vi "ClimbExecute_SIM.vi"(8 "error in (no error)":errorcluster, 11 "Inputs":T3) -> (0 "error out":errorcluster, 2 "InfoOutput":T1, 3 "Outputs":T2)   [LabVIEW 2023]
uses:
  <vilib>/Rock Robotics/WPI/ThirdParty/JAS_Junk/TrajLib/Timer_New.vi
  <vilib>/Rock Robotics/WPI/ThirdParty/JAS_Junk/TrajLib/VI/BoolCmd_Recv_Internal.vi
  <vilib>/Rock Robotics/WPI/ThirdParty/JAS_Junk/TrajLib/VI/BoolCmd_ObtainQueue.vi
  <vilib>/Rock Robotics/Network Tables/NT Write Number.vi
  <vilib>/Utility/semaphor.llb/Obtain Semaphore Reference.vi
  <vilib>/Rock Robotics/WPI/ThirdParty/JAS_Junk/TrajLib/Timer_Reset.vi
  <vilib>/Rock Robotics/WPI/ThirdParty/JAS_Junk/TrajLib/Timer_Start.vi
  <vilib>/Rock Robotics/WPI/ThirdParty/JAS_Junk/TrajLib/Timer_Stop.vi
  <vilib>/Rock Robotics/WPI/ThirdParty/JAS_Junk/TrajLib/Timer_HasPeriodPassedOnce.vi
  <vilib>/Rock Robotics/Network Tables/NT Write Boolean.vi
  <vilib>/Rock Robotics/WPI/ThirdParty/JAS_Junk/TrajLib/Trajectory_Library.lvlib
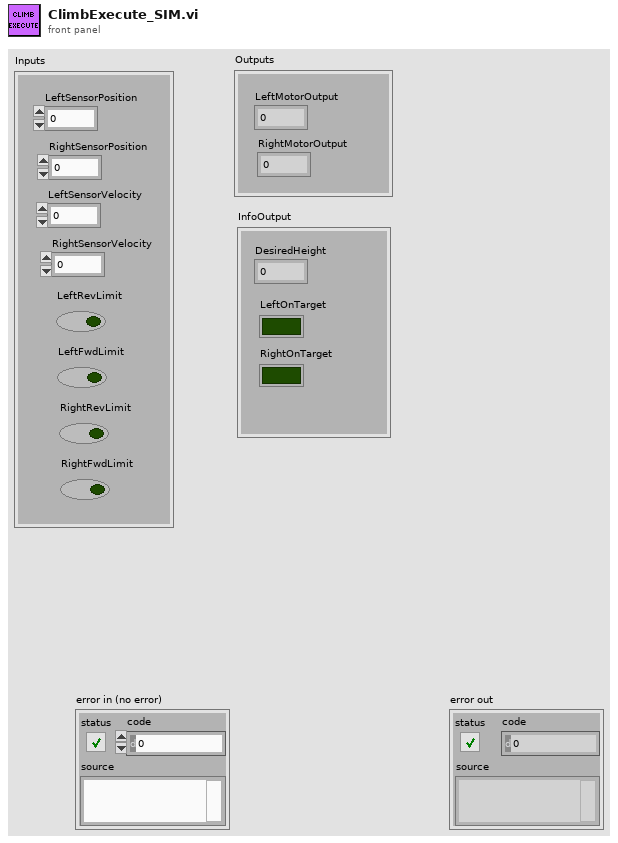
[diagram p1: front panel]
types:
  T1 = cluster{"DesiredHeight":dbl, "LeftOnTarget":bool, "RightOnTarget":bool}
  T2 = cluster{"LeftMotorOutput":dbl, "RightMotorOutput":dbl}
  T3 = cluster{"LeftSensorPosition":dbl, "RightSensorPosition":dbl, "LeftSensorVelocity":dbl, "RightSensorVelocity":dbl, "LeftRevLimit":bool, "LeftFwdLimit":bool, "RightRevLimit":bool, "RightFwdLimit":bool}
  T4 = typedef "Trajectory_Library.lvlib/PosCtrl_Tuning_Type.ctl" = cluster{"Slope":dbl, "Offset":dbl, "Error Deadband":dbl, "At Reference Count":i32, "Negate Output":bool, "Max Allowd Position":dbl, "Min Allowd Position":dbl}
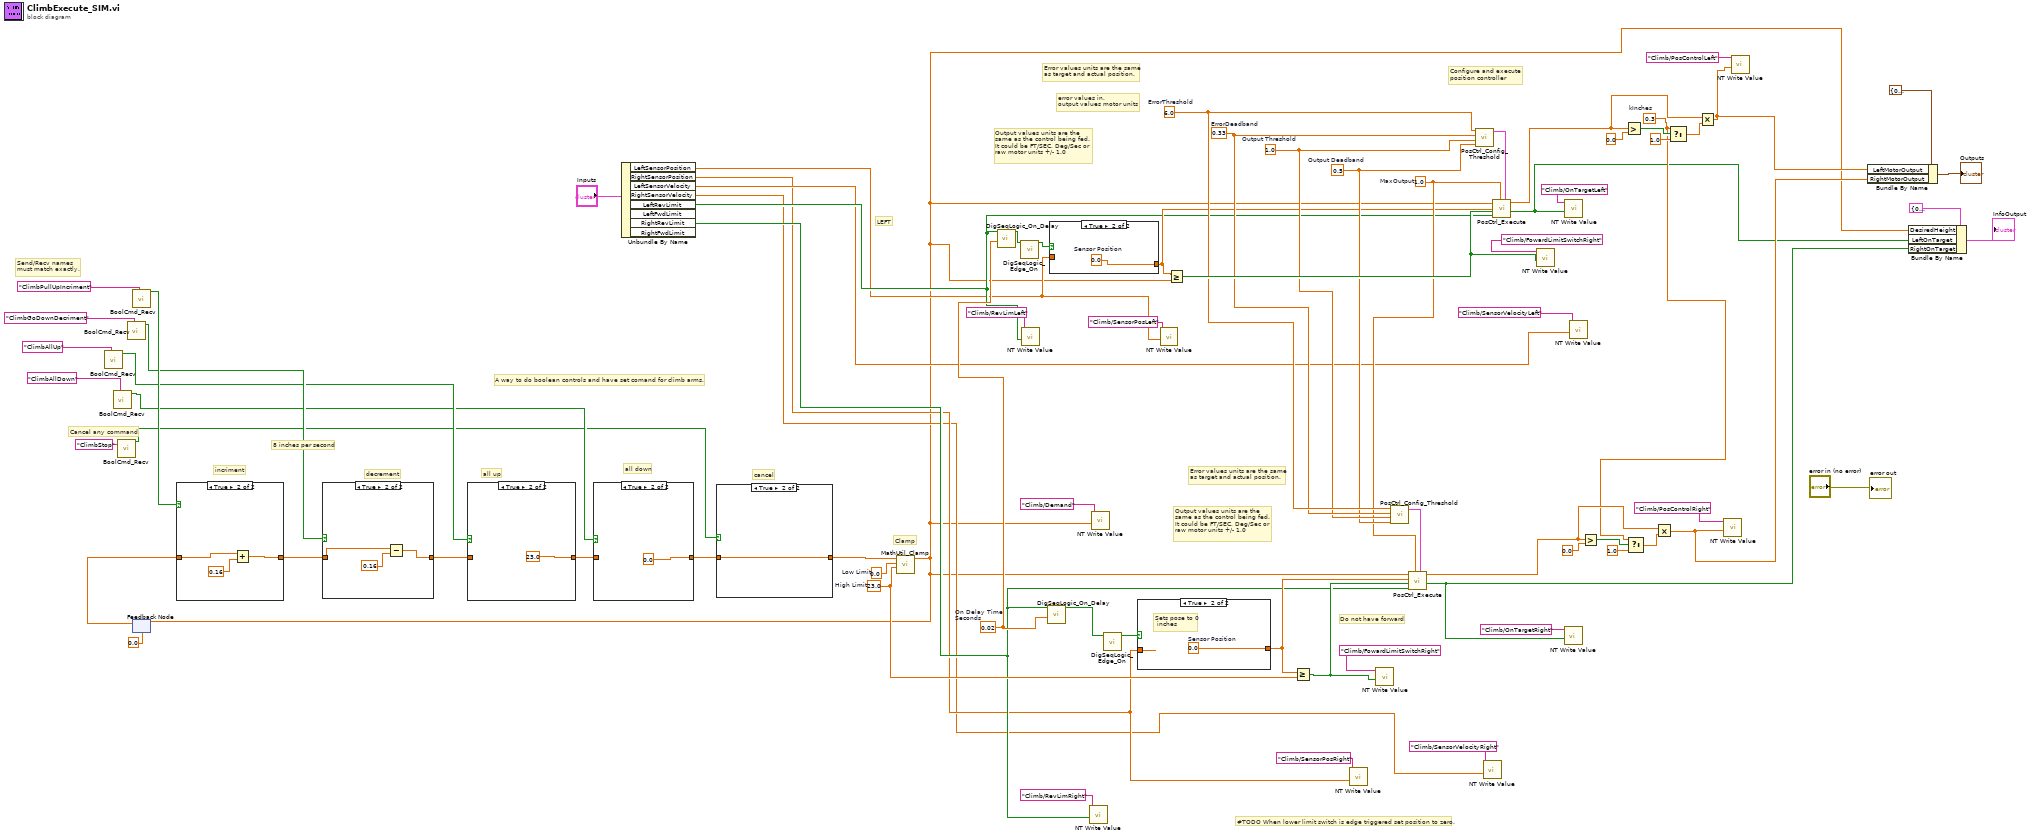
[diagram p0: block diagram]
diagram:
  w17 = 0.3  # kInches
  w32 = 0.02  # On Delay Time Seconds
  w45 = 23.0  # High Limit
  w54 = 0.0  # Low Limit
  w34 = 1.0  # MaxOutput
  w38 = 6.0  # ErrorThreshold
  w37 = 0.33  # ErrorDeadband
  w36 = 1.0  # Output Threshold
  w35 = 0.5  # Output Deadband
  # "LEFT"
  # "#TODO When lower limit switch is edge triggered set position to zero."
  # "cancel"
  # "Clamp"
  # "8 inches per second"
  # "all down"
  # "all up"
  # "decrement"
  # "incriment"
  # "Cancel any command"
  # "Send/Recv names\nmust match exactly."
  # "A way to do boolean controls and have set comand for climb arms."
  # "error values in.\noutput values motor units"
  # "Do not have forward"
  # "Output values units are the\nsame as the control being fed.  \nIt could be FT/SEC, Deg/Sec or\nraw motor units +/- 1.0"
  # "Error values units are the same \nas target and actual position."
  # "Output values units are the\nsame as the control being fed.  \nIt could be FT/SEC, Deg/Sec or\nraw motor units +/- 1.0"
  # "Error values units are the same \nas target and actual position."
  # "Configure and execute \nposition controller"
  n1 = call <vilib>:"BoolCmd_Recv.vi"("Command Name"="ClimbAllUp") -> ("New Request"=w49:bool)  [unwired: 9 in, 1 out]
  n2 = call <vilib>:"BoolCmd_Recv.vi"("Command Name"="ClimbAllDown") -> ("New Request"=w48:bool)  [unwired: 9 in, 1 out]
  n3 = call <vilib>:"BoolCmd_Recv.vi"("Command Name"="ClimbStop") -> ("New Request"=w47:bool)  [unwired: 9 in, 1 out]
  n4 = call <vilib>:"BoolCmd_Recv.vi"("Command Name"="ClimbGoDownDecriment") -> ("New Request"=w50:bool)  [unwired: 9 in, 1 out]
  n5 = call <vilib>:"BoolCmd_Recv.vi"("Command Name"="ClimbPullUpIncriment") -> ("New Request"=w51:bool)  [unwired: 9 in, 1 out]
  n6 = feedback #1(0.0 ("false")) -> (w58:dbl)
  n7 = case shown="True" w51 {
    tunnel: w58 -> [w77 w80]
    tunnel: [w77 w78] -> w57
    frame False {
    }
    frame True {
      n8 = Add(x=w80, y=0.16) -> (x+y=w78:dbl)
    }
  }
  n9 = case shown="True" w50 {
    tunnel: w57 -> [w81 w83]
    tunnel: [w81 w82] -> w56
    frame False {
    }
    frame True {
      n10 = Subtract(x=w83, y=0.16) -> (x-y=w82:dbl)
    }
  }
  n11 = case shown="True" w49 {
    tunnel: w56 -> [w85 _]
    tunnel: [w85 23.0 ("y")] -> w55
    frame False {
    }
    frame True {
    }
  }
  n12 = case shown="True" w48 {
    tunnel: w55 -> [w87 _]
    tunnel: [w87 0.0 ("y")] -> w53
    frame False {
    }
    frame True {
    }
  }
  n13 = Unbundle By Name("Inputs") -> ("LeftSensorPosition"=w14:dbl, "RightSensorPosition"=w8:dbl, "LeftSensorVelocity"=w13:dbl, "RightSensorVelocity"=w7:dbl, "LeftRevLimit"=w15:bool, "RightRevLimit"=w9:bool)  [unwired: 2 out]
  n14 = case shown="True" w47 {
    tunnel: w53 -> [w89 w90]
    tunnel: [w89 w90] -> w52
    frame False {
    }
    frame True {
    }
  }
  n15 = call <vilib>:"MathUtil_Clamp.vi"("High Limit"=w45, "Low Limit"=w54, "Value"=w52) -> ("Result"=w1:dbl)  [unwired: 8 in]
  n16 = feedback-in #1(w1) -> ()
  n17 = call <vilib>:"DigSeqLogic_On_Delay.vi"("Delay"=w32, "Input"=w15) -> ("Output"=w31:bool)  [unwired: 8 in, 1 out]
  n18 = call <vilib>:"DigSeqLogic_Edge_On.vi"("Input"=w31) -> ("On Edge"=w30:bool)  [unwired: 10 in]
  n19 = call-poly <vilib>:"NT Write Value.vi"("value"=w15, "name"="Climb/RevLimLeft") -> ()  [unwired: 9 in, 1 out]
  n20 = call <vilib>:"DigSeqLogic_On_Delay.vi"("Delay"=w32, "Input"=w9) -> ("Output"=w40:bool)  [unwired: 8 in, 1 out]
  n21 = case shown="True" w30 {
    tunnel: w14 -> [w91 _]
    tunnel: [w91 w92] -> w29
    frame False {
    }
    frame True {
      w92 = 0.0  # Sensor Position
    }
  }
  n22 = call-poly <vilib>:"NT Write Value.vi"("value"=w9, "name"="Climb/RevLimRight") -> ()  [unwired: 9 in, 1 out]
  n23 = call-poly <vilib>:"NT Write Value.vi"("value"=w1, "name"="Climb/Demand") -> ()  [unwired: 9 in, 1 out]
  n24 = call <vilib>:"DigSeqLogic_Edge_On.vi"("Input"=w40) -> ("On Edge"=w33:bool)  [unwired: 10 in]
  n25 = case shown="True" w33 {
    tunnel: w8 -> [w93 _]
    tunnel: [w93 w94] -> w39
    frame False {
    }
    frame True {
      w94 = 0.0  # Sensor Position
      # "Sets pose to 0\n inches"
    }
  }
  n26 = call-poly <vilib>:"NT Write Value.vi"("value"=w14, "name"="Climb/SensorPosLeft") -> ()  [unwired: 9 in, 1 out]
  n27 = Greater Or Equal?(x=w29, y=w1) -> (x >= y?=w41:bool)
  n28 = Greater Or Equal?(x=w39, y=w45) -> (x >= y?=w43:bool)
  n29 = call-poly <vilib>:"NT Write Value.vi"("value"=w8, "name"="Climb/SensorPosRight") -> ()  [unwired: 9 in, 1 out]
  n30 = call-poly <vilib>:"NT Write Value.vi"("value"=w43, "name"="Climb/FowardLimitSwitchRight") -> ()  [unwired: 9 in, 1 out]
  n31 = call <vilib>:"PosCtrl_Config_Threshold.vi"("Output Deadband"=w35, "Output Threshold"=w36, "ErrorDeadband"=w37, "ErrorThreshold"=w38) -> ("PosCtrl_Config_Params"=w66:T4)  [unwired: 7 in]
  n32 = call <vilib>:"PosCtrl_Execute.vi"("PosCtrl_Config_Params"=w66, "MaxOutput"=w34, "Rev Limit Switch"=w9, "Fwd Limit Switch"=w43, "CurrentPosition"=w39, "TargetPosition"=w1) -> ("OnTarget"=w2:bool, "Output"=w18:dbl)  [unwired: 3 in, 1 out]
  n33 = call <vilib>:"PosCtrl_Config_Threshold.vi"("Output Deadband"=w35, "Output Threshold"=w36, "ErrorDeadband"=w37, "ErrorThreshold"=w38) -> ("PosCtrl_Config_Params"=w76:T4)  [unwired: 7 in]
  n34 = call-poly <vilib>:"NT Write Value.vi"("value"=w7, "name"="Climb/SensorVelocityRight") -> ()  [unwired: 9 in, 1 out]
  n35 = call <vilib>:"PosCtrl_Execute.vi"("PosCtrl_Config_Params"=w76, "MaxOutput"=w34, "Rev Limit Switch"=w15, "Fwd Limit Switch"=w41, "CurrentPosition"=w29, "TargetPosition"=w1) -> ("OnTarget"=w3:bool, "Output"=w24:dbl)  [unwired: 3 in, 1 out]
  n36 = call-poly <vilib>:"NT Write Value.vi"("value"=w41, "name"="Climb/FowardLimitSwitchRight") -> ()  [unwired: 9 in, 1 out]
  n37 = call-poly <vilib>:"NT Write Value.vi"("value"=w2, "name"="Climb/OnTargetRight") -> ()  [unwired: 9 in, 1 out]
  n38 = call-poly <vilib>:"NT Write Value.vi"("value"=w3, "name"="Climb/OnTargetLeft") -> ()  [unwired: 9 in, 1 out]
  n39 = call-poly <vilib>:"NT Write Value.vi"("value"=w13, "name"="Climb/SensorVelocityLeft") -> ()  [unwired: 9 in, 1 out]
  n40 = Greater?(x=w18, y=0.0) -> (0:w22:bool)
  n41 = Greater?(x=w24, y=0.0) -> (0:w27:bool)
  n42 = Select(t=w17, s=w22, f=1.0) -> (s? t:f=w20:dbl)
  n43 = Multiply(x=w18, y=w20) -> (x*y=w6:dbl)
  n44 = Select(t=w17, s=w27, f=1.0) -> (s? t:f=w25:dbl)
  n45 = Multiply(x=w24, y=w25) -> (x*y=w10:dbl)
  n46 = call-poly <vilib>:"NT Write Value.vi"("value"=w6, "name"="Climb/PosControlRight") -> ()  [unwired: 9 in, 1 out]
  n47 = call-poly <vilib>:"NT Write Value.vi"("value"=w10, "name"="Climb/PosControlLeft") -> ()  [unwired: 9 in, 1 out]
  n48 = Bundle By Name(cluster=T2 {"LeftMotorOutput"=0.0, "RightMotorOutput"=0.0} ("Outputs"), "LeftMotorOutput"=w10, "RightMotorOutput"=w6) -> (→"Outputs":T2)
  n49 = Bundle By Name(cluster=T1 {"DesiredHeight"=0.0, "LeftOnTarget"=FALSE, "RightOnTarget"=FALSE} ("InfoOutput"), "DesiredHeight"=w1, "LeftOnTarget"=w3, "RightOnTarget"=w2) -> (→"InfoOutput":T1)
  "error out" <- "error in (no error)"
